vi "Instrument Do Core.vi"(8 "error in (no error)":errorcluster, 9 "Instrument in":refnum<class "Instrument Driver.lvclass">, 10 "Actor in":refnum<class "Actor.lvclass">, 11 "DMM Triggered Measure Msg in":refnum<class "DMM Triggered Measure Msg.lvclass">) -> (0 "error out":errorcluster, 1 "Instrument out":refnum<class "Instrument Driver.lvclass">, 2 "Actor out":refnum<class "Actor.lvclass">, 3 "DMM Triggered Measure Msg out":refnum<class "DMM Triggered Measure Msg.lvclass">, 5 "Data":refnum<class "Data.lvclass">)   [LabVIEW 2020, in "DMM Msg.lvlib" / "DMM Triggered Measure Msg.lvclass"]
doc: "Perform a measurement using the DMM and returning the results in a DMM Measurement Data class."
uses:
  DMM Triggered Measure Msg.lvclass
  PPL/HDH.Actor Framework.Core.Actor.lvlibp/1abvi3w/vi.lib/ActorFramework/Actor/Actor.lvclass
  PPL/HDH.Data.Generic.lvlibp/Data.lvclass
  PPL/HDH.Actor Framework.Core.Instrument Driver.lvlibp/Instrument Driver/Instrument Driver.lvclass
  PPL/HDH.Driver.DMM.lvlibp/DMM Driver.lvclass
  C:/Current projects/WS/PPL/HDH.Actor Framework.Core.Instrument Driver.lvlibp/Instrument Driver/Instrument Driver.lvclass
  Data/DMM Measurement Data/DMM Measurement Data.lvclass
  C:/Current projects/WS/PPL/HDH.Data.Generic.lvlibp/Data.lvclass
  DMM Triggered Measure Msg.lvclass/DMM Triggered Measure Msg.ctl
  Data/DMM Measurement Data/DMM Measurement Data.lvclass/DMM Measurement Data.ctl
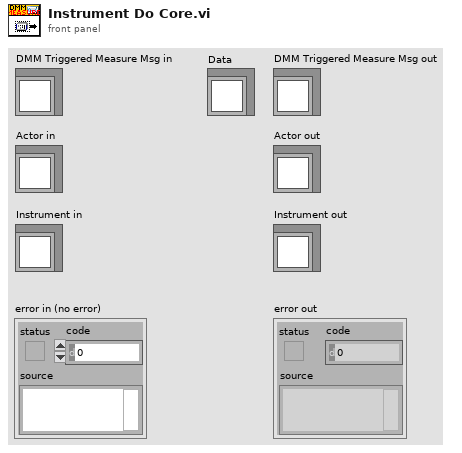
[diagram p1: front panel]
types:
  T1 = typedef "HDH.Driver.DMM.lvlibp/Ctl_Function.ctl" = enum8{"DC Volts", "AC Volts", "DC Current", "AC Current", "2-wire Resistance", "4-wire Resistance", "Diode", "Frequency", "Period", "AC Volts DC Coupled", "Capacitance", "Inductance", "Temperature"}
  T2 = typedef "HDH.Driver.DMM.lvlibp/Ctl_DigitResolution.ctl" = enum8{"3½", "4½", "5½", "6½", "7½"}
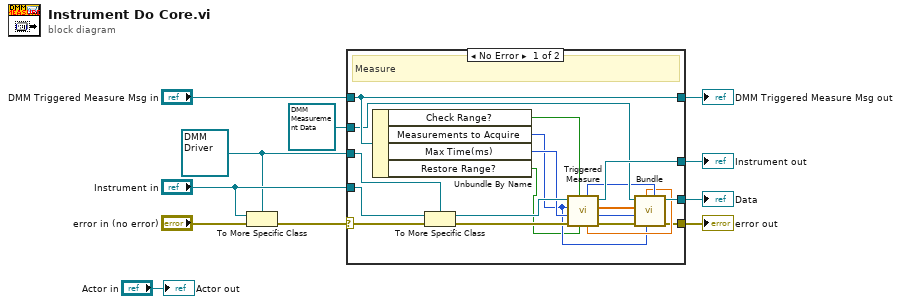
[diagram p0: block diagram]
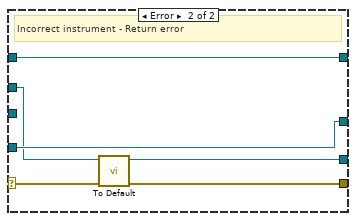
[diagram p2: hidden frame]
diagram:
  w5 = refnum<class "DMM Driver.lvclass"> refnum ("HDH.Driver.DMM.lvlibp:DMM Driver.lvclass")
  n1 = To More Specific Class(target class=w5, reference="Instrument in", error in="error in (no error)") -> (error out=w10:errorcluster)  [unwired: 1 out]
  n2 = case shown="No Error" w10 {
    selector: w10 -> [w30 w32]
    tunnel: [w14 w31] -> w3
    tunnel: [w27 w36] -> w9
    tunnel: "DMM Triggered Measure Msg in" -> [w27 w36]
    tunnel: [w24 w35] -> w7
    tunnel: "Instrument in" -> [w29 w35]
    tunnel: w5 -> [w28 _]
    tunnel: [w21 w33] -> w2
    tunnel: refnum<class "DMM Measurement Data.lvclass"> refnum ("DMM Measurement Data in") -> [w22 w34]
    frame No Error {
      # "Measure"
      n3 = Unbundle By Name(w27) -> ("Check Range?"=w12:bool, "Measurements to Acquire"=w16:i32, "Max Time(ms)"=w23:i32, "Restore Range?"=w13:bool)
      n4 = To More Specific Class(target class=w28, reference=w29, error in=w30) -> (specific class reference=w25:refnum<class "DMM Driver.lvclass">, error out=w26:errorcluster)
      n5 = call "Triggered Measure.vi"("Restore Range if Checked?(T)"=w13, "Check Range?(T)"=w12, "error in (no error)"=w26, "Max Time (-1ms)"=w23, "Measurements to Acquire(1)"=w16, "DMM Driver in"=w25) -> ("error out"=w15:errorcluster, "Function"=w18:T1, "Measurements"=w19:dbl[], "DMM Driver out"=w24:refnum<class "DMM Driver.lvclass">, "Range"=w17:dbl, "Digit Resolution(5½)"=w20:T2)
      n6 = call "Bundle.vi"("Digit Resolution"=w20, "Target Measurement Count"=w16, "Range"=w17, "error in (no error)"=w15, "Function"=w18, "Measurements"=w19, "DMM Measurement Data in"=w22) -> ("error out"=w14:errorcluster, "DMM Measurement Data out"=w21:refnum<class "DMM Measurement Data.lvclass">)  [unwired: 3 in]
    }
    frame Error {
      # "Incorrect instrument - Return error"
      n7 = call-dynamic "To Default.vi"("error in (no error)"=w32, "Data in"=w34) -> ("error dub"=w31:errorcluster, "Data out"=w33:refnum<class "DMM Measurement Data.lvclass">)  [unwired: 8 in]
    }
  }
  "error out" <- w3
  "DMM Triggered Measure Msg out" <- w9
  "Instrument out" <- w7
  "Data" <- w2
  "Actor out" <- "Actor in"
